vi "test_Queue.vi"() -> ()   [LabVIEW 2014]
doc: "Testuje działanie kolejki Queue"
uses:
  Client.ctl
  LukiBrary.lvlib
panel:
  out "People":T1[](array[typedef])
  out "usunięty":T1
  in  "lambda":dbl=0.1 format="%#_13g"
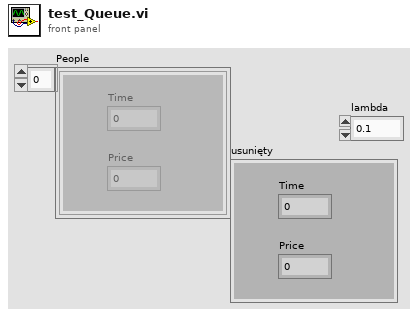
[diagram p1: front panel]
types:
  T1 = typedef "LukiBrary.lvlib/Client.ctl" = cluster{"Time":dbl, "Price":dbl}
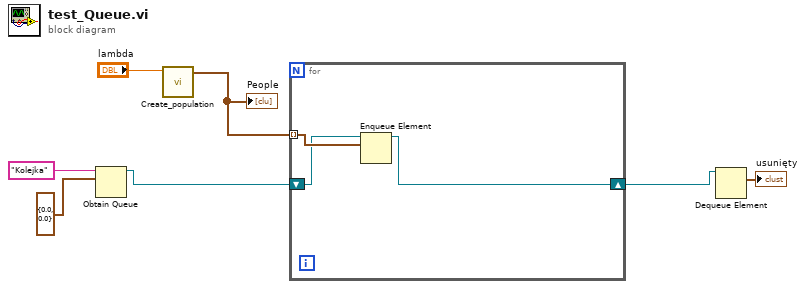
[diagram p0: block diagram]
diagram:
  n1 = Obtain Queue(name (unnamed)="Kolejka", element data type=T1 {"Time"=0.0, "Price"=0.0} ("Client")) -> (queue out=w3:refnum<queue>)  [unwired: 3 in, 2 out]
  n2 = call "Create_population.vi"("lambda"="lambda") -> ("People"=w4:T1[])  [unwired: 10 in]
  "People" <- w4
  n3 = for {
    tunnel: w4 -> [w10] mode=indexing
    shift-right: [w8] -> w2
    shift-left: w3 -> [w9]
    n4 = Enqueue Element(queue=w9, element=w10) -> (queue out=w8:refnum<queue>)  [unwired: 2 in, 2 out]
  }
  n5 = Dequeue Element(queue=w2) -> (element=→"usunięty":T1)  [unwired: 2 in, 3 out]
